vi "Stop-plant.vi"(8 "error in (no error)":errorcluster, 10 "Plant VI path":path=path "C:/ni-rt/startup/Plant1.vi", 11 "Machine IP Address":string="193.0.0.2") -> (0 "error out":errorcluster)   [LabVIEW 2016]
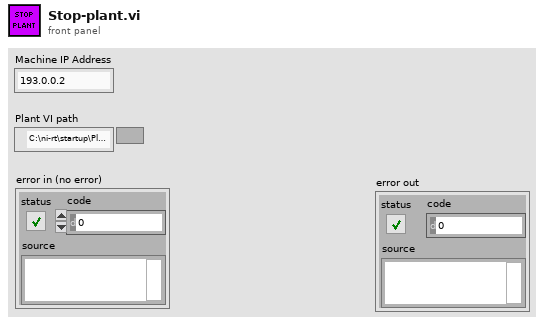
[diagram p1: front panel]
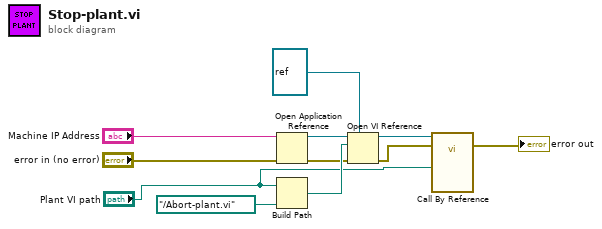
[diagram p0: block diagram]
diagram:
  n1 = Open Application Reference(8:"error in (no error)", 11:"Machine IP Address") -> (0:w3:errorcluster, 3:w5:refnum<vi>)  [unwired: 2 in]
  n2 = Build Path(base path="Plant VI path", name or relative path=path "../Abort-plant.vi") -> (appended path=w10:path)
  n3 = Open VI Reference(type specifier VI Refnum (for type only)=refnum<vi> refnum, application reference (local)=w5, vi path=w10, error in (no error)=w3) -> (vi reference=w8:refnum<vi>, error out=w6:errorcluster)  [unwired: 2 in]
  n4 = call-by-ref "?"(reference=w8, error in=w6, "Plant VI path"="Plant VI path") -> (error out=→"error out":errorcluster)  [unwired: 10 in, 2 out]
